vi "Configure Q-Switch Delay.vi"(7 "Q-switch (primary)":u16(ring)=1 items=["primary"=1, "secondary"=2], 8 "error in (no error)":errorcluster, 11 "Lotis in":refnum<class "PL Lotis TII LS.lvclass">) -> (0 "error out":errorcluster, 3 "Lotis out":refnum<class "PL Lotis TII LS.lvclass">)   [LabVIEW 2015, in "PL Lotis TII LS.lvclass"]
doc: "Configures Q-switch delay."
uses:
  PL Lotis TII LS.lvclass
panel:
  in  "delay, ns":u32
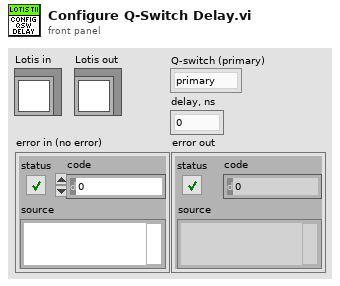
[diagram p1: front panel]
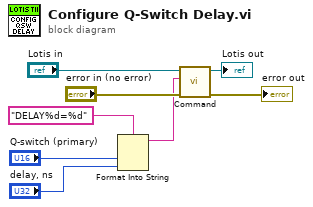
[diagram p0: block diagram]
diagram:
  n1 = Format Into String(format string="DELAY%d=%d" ("command"), "Q-switch (primary)", "delay, ns") -> (resulting string=w3:string)  [unwired: 2 in, 1 out]
  n2 = call "Command.vi"("error in (no error)"="error in (no error)", "command"=w3, "Lotis in"="Lotis in") -> ("error out"=→"error out":errorcluster, "Lotis out"=→"Lotis out":refnum<class "PL Lotis TII LS.lvclass">)  [unwired: 6 in, 1 out]
